vi "Smooth Turret.vi"(11 "tx":dbl) -> (3 "smoothed tx":dbl)   [LabVIEW 2019]
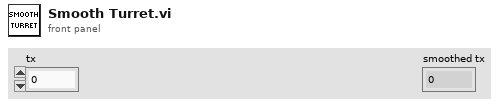
[diagram p1: front panel]
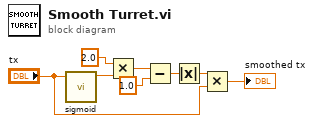
[diagram p0: block diagram]
diagram:
  n1 = call "sigmoid.vi"("x"="tx") -> ("sigmoid(x)"=w8:dbl)  [unwired: 10 in]
  n2 = Multiply(x=2.0, y=w8) -> (x*y=w6:dbl)
  n3 = Subtract(x=w6, y=1.0) -> (x-y=w2:dbl)
  n4 = Absolute Value(x=w2) -> (abs(x)=w1:dbl)
  n5 = Multiply(x=w1, y="tx") -> (x*y=→"smoothed tx":dbl)
